vi "KObjTemplate-From Variant.vi"(0 "Obj in":refnum<class "KObject.lvclass">, 7 "Variant":variant, 9 "Prefix":string, 11 "error in (no error)":errorcluster) -> (4 "Obj out":refnum<class "KObject.lvclass">, 15 "error out":errorcluster)   [LabVIEW 2015]
uses:
  KObject Class/KObject.lvclass
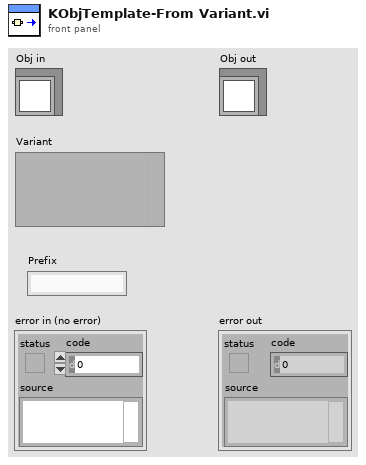
[diagram p1: front panel]
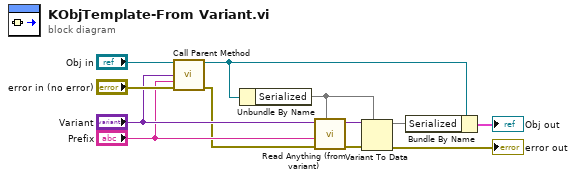
[diagram p0: block diagram]
diagram:
  n1 = call-parent "Call Parent Method"("TTLDevice in"="Obj in", "Variant"="Variant", "Prefix"="Prefix", "error in (no error)"="error in (no error)") -> ("TTLDevice out"=w3:refnum<class "TTLWaterDelivery.lvclass">, "error out"=w4:errorcluster)  [unwired: 10 in]
  n2 = Unbundle By Name(w3) -> ("Serialized"=w8)
  n3 = call "Read Anything (from variant).vi"("Type of Anything"=w8, "Error In"=w4, "Prefix"="Prefix", "Variant Database"="Variant") -> ("Error Out"=w9:errorcluster, "Anything"=w10:variant)  [unwired: 5 in, 1 out]
  n4 = Variant To Data(error in=w9, type=w8, Variant=w10) -> (data=w7, error out=→"error out":errorcluster)
  n5 = Bundle By Name(cluster=w3, "Serialized"=w7) -> (→"Obj out":cluster{})
